vi "phforge Script.vi"(8 "Error in":errorcluster, 9 "Output File Path":path, 10 "HDF5 File Path":path, 11 "Metadata File Path":path) -> (0 "Error out":errorcluster, 1 "Return Code":i32, 2 "Standard Error":string, 3 "Standard Output":string)   [LabVIEW 2010]
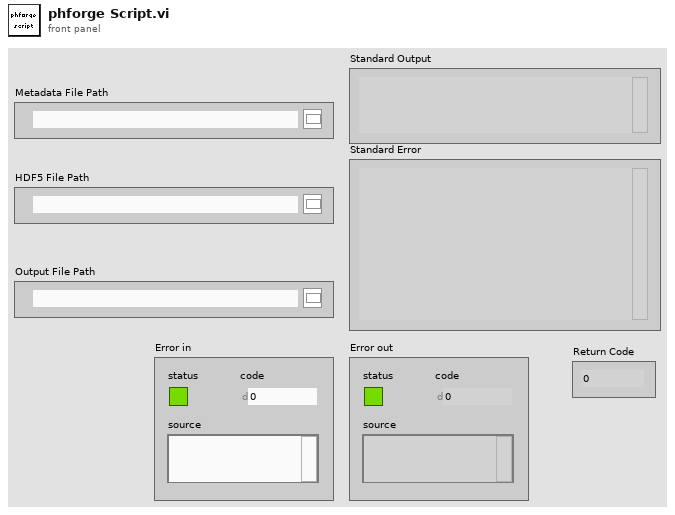
[diagram p1: front panel]
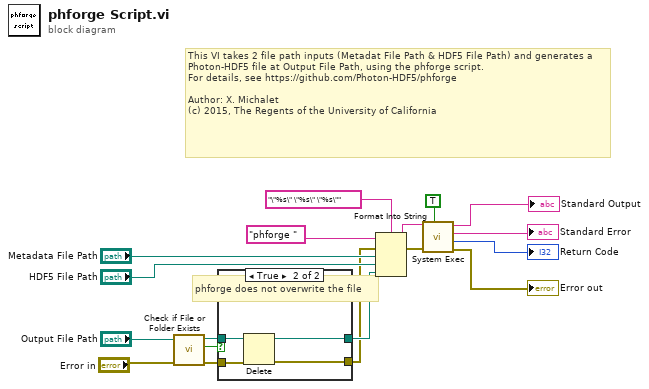
[diagram p0: block diagram]
diagram:
  # "This VI takes 2 file path inputs (Metadat File Path & HDF5 File Path) and generates a Photon-HDF5 file at Output File Path, using the phforge script.\nFor details, see https://github.com/Photon-HDF5/phforge\n\nAuthor: X. Michalet\n(c) 2015, The Regents of the University of California"
  n1 = call <vilib>:"Check if File or Folder Exists.vi"("error in (no error)"="Error in", "path"="Output File Path") -> ("error out"=w2:errorcluster, "file or folder exists?"=w5:bool, "dup path"=w4:path)  [unwired: 7 in]
  n2 = case shown="True" w5 {
    tunnel: w4 -> [w20 w24]
    tunnel: [w20 w22] -> w3
    tunnel: w2 -> [w19 w23]
    tunnel: [w19 w21] -> w1
    frame False {
    }
    frame True {
      # "phforge does not overwrite the file"
      n3 = Delete(path (use dialog)=w24, error in=w23) -> (deleted path=w22:path, error out=w21:errorcluster)  [unwired: 3 in, 1 out]
    }
  }
  n4 = Format Into String(format string="\"%s\" \"%s\" \"%s\"" ("command line"), initial string="phforge ", error in=w1, "Metadata File Path", "HDF5 File Path", w3) -> (resulting string=w9:string, error out=w12:errorcluster)
  n5 = call <vilib>:"System Exec.vi"("wait until completion? (T)"=TRUE, "error in (no error)"=w12, "command line"=w9) -> ("error out"=→"Error out":errorcluster, "return code"=→"Return Code":i32, "standard error"=→"Standard Error":string, "standard output"=→"Standard Output":string)  [unwired: 5 in]
